vi "Client LNA Started.vi"(8 "error in (no error)":errorcluster, 11 "Client Controller in":refnum<class "Client Controller.lvclass">) -> (0 "error out":errorcluster, 3 "Client Controller out":refnum<class "Client Controller.lvclass">)   [LabVIEW 2016, in "Client Controller.lvlib" / "Client Controller.lvclass"]
uses:
  Client Controller.lvclass
  Client Controller.lvclass/Client Controller.ctl
  <vilib>/ActorFramework/Message Enqueuer/Message Enqueuer.lvclass
  <vilib>/NI/Actors/Linked Network Actor/Linked Network Actor Messages/Disconnect Msg/Disconnect Msg.lvclass
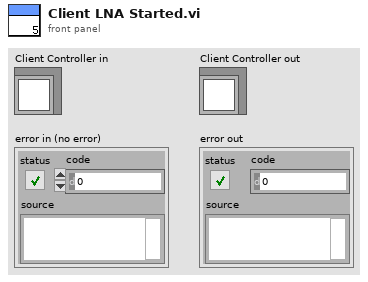
[diagram p1: front panel]
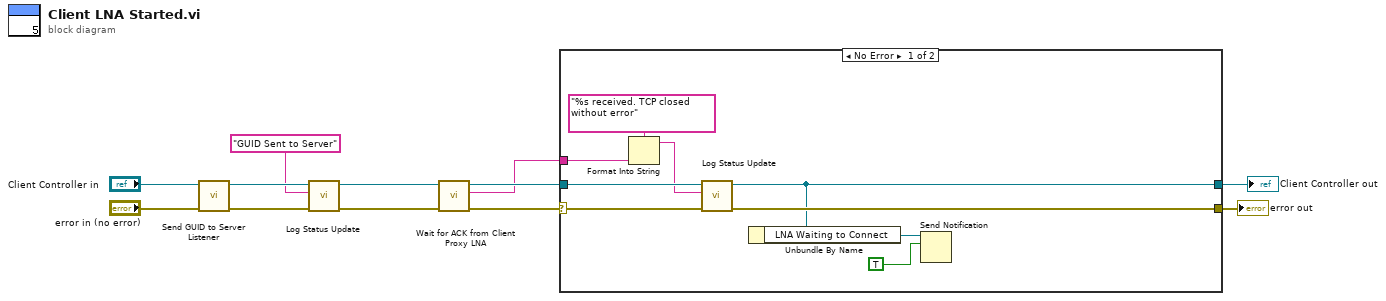
[diagram p0: block diagram]
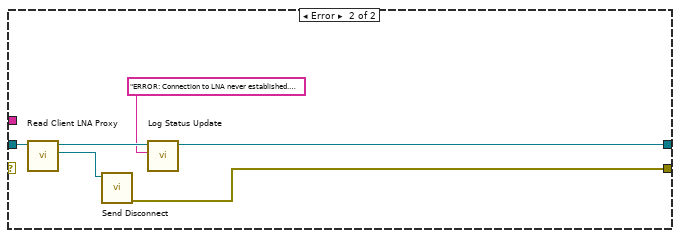
[diagram p2: hidden frame]
diagram:
  n1 = call "Send GUID to Server Listener.vi"("error in (no error)"="error in (no error)", "Client Controller in"="Client Controller in") -> ("error out"=w5:errorcluster, "Client Controller out"=w12:refnum<class "Client Controller.lvclass">)  [unwired: 8 in]
  n2 = call-dynamic "Log Status Update.vi"("error in (no error)"=w5, "String"="GUID Sent to Server", "Controller in"=w12) -> ("error out"=w3:errorcluster, "Controller out"=w4:refnum<class "Client Controller.lvclass">)  [unwired: 7 in]
  n3 = call "Wait for ACK from Client Proxy LNA.vi"("error in (no error)"=w3, "Client Controller in"=w4) -> ("error out"=w9:errorcluster, "data out"=w1:string, "Client Controller out"=w2:refnum<class "Client Controller.lvclass">)  [unwired: 7 in]
  n4 = case shown="No Error" w9 {
    selector: w9 -> [w19 _]
    tunnel: w2 -> [w21 w22]
    tunnel: [w15 w25] -> w10
    tunnel: [w20 w23] -> w11
    tunnel: w1 -> [w17 _]
    frame No Error {
      n5 = Format Into String(format string="%s received. TCP closed without error" ("String"), w17) -> (resulting string=w16:string)  [unwired: 2 in, 1 out]
      n6 = call-dynamic "Log Status Update.vi"("error in (no error)"=w19, "String"=w16, "Controller in"=w21) -> ("error out"=w20:errorcluster, "Controller out"=w15:refnum<class "Client Controller.lvclass">)  [unwired: 7 in]
      n7 = Unbundle By Name(w15) -> ("LNA Waiting to Connect"=w14:refnum<notifier>)
      n8 = Send Notification(notification=TRUE, notifier=w14) -> ()  [unwired: 1 in, 2 out]
    }
    frame Error {
      n9 = call "Read Client LNA Proxy.vi"("Client Controller in"=w22) -> ("Actor Framework:Message Enqueuer"=w24:refnum<class "Message Enqueuer.lvclass">, "Client Controller out"=w27:refnum<class "Client Controller.lvclass">)  [unwired: 8 in, 1 out]
      n10 = call <vilib>:"Send Disconnect.vi"("Message Enqueuer"=w24) -> ("error out"=w23:errorcluster)  [unwired: 9 in, 1 out]
      n11 = call-dynamic "Log Status Update.vi"("String"="ERROR: Connection to LNA never established. Shutting down client LNA and retrying", "Controller in"=w27) -> ("Controller out"=w25:refnum<class "Client Controller.lvclass">)  [unwired: 8 in, 1 out]
    }
  }
  "error out" <- w11
  "Client Controller out" <- w10
